vi "NXT_HINDBRAIN Get Sensor Data.vi"(3 "_motorCommands":T1={"_rudderCommand"=7, "_propCommand"=7, "_irServoCommand"=7}, 4 "_sensorData":T2, 5 "NXT":T4) -> (1 "_sensorData":T2)   [LabVIEW 2012, in "Tugboat.lvrbt"]
uses:
  Tugboat.lvrbt
  sensorData_t.ctl
  irData_t.ctl
  <vilib>/NXT/Subs/LVHSConnector.ctl
  motorCommands_t.ctl
  <vilib>/NXT/Block Support/NXT_ButtonSelector.ctl
  <vilib>/NXT/Block Support/NXT_InputPort.ctl
  <vilib>/NXT/Block Support/NXT_TimerIndex.ctl
panel:
  # "L\nE\nF\nT"
  # "C\nE\nN\nT\nE\nR"
  # "R\nI\nG\nH\nT"
  # "L\nE\nF\nT"
  # "C\nE\nN\nT\nE\nR"
  # "R\nI\nG\nH\nT"
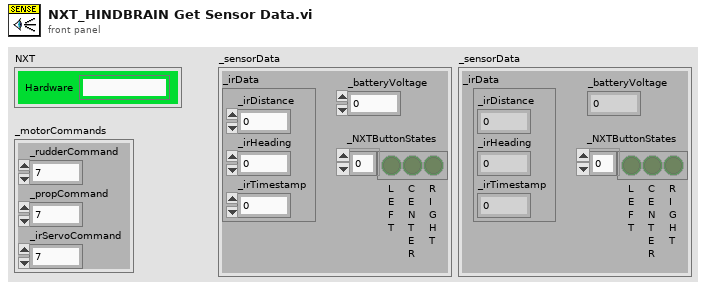
[diagram p1: front panel]
types:
  T1 = typedef "motorCommands_t.ctl" = cluster{"_rudderCommand":i8, "_propCommand":i8, "_irServoCommand":i8}
  T2 = typedef "sensorData_t.ctl" = cluster{"_irData":T3, "_batteryVoltage":i32, "_NXTButtonStates":bool[]}
  T3 = typedef "irData_t.ctl" = cluster{"_irDistance":i32, "_irHeading":i32, "_irTimestamp":u32}
  T4 = typedef "LVHSConnector.ctl" = cluster{"Hardware":string, "Flattened String":string}
  T5 = typedef "NXT_TimerIndex.ctl" = u8
  T6 = typedef "NXT_InputPort.ctl" = u8
  T7 = typedef "NXT_ButtonSelector.ctl" = u16
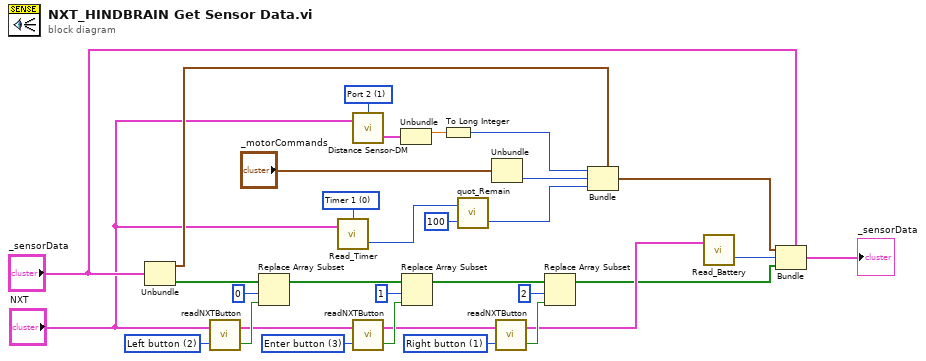
[diagram p0: block diagram]
diagram:
  w7 = T5 0 items=["Timer 1", "Timer 2", "Timer 3"] ("Timer (Timer 1)")
  w13 = T6 1 items=["Port 1", "Port 2", "Port 3", "Port 4"] ("Input Port")
  w19 = T7 1 items=["Enter button"=3, "Left button"=2, "Right button"=1] ("Button (Enter button)")
  w22 = T7 3 items=["Enter button"=3, "Left button"=2, "Right button"=1] ("Button (Enter button)")
  w26 = T7 2 items=["Enter button"=3, "Left button"=2, "Right button"=1] ("Button (Enter button)")
  n1 = Unbundle("_sensorData") -> ("_irData"=w11:T3, "_NXTButtonStates"=w29:bool[])  [unwired: 1 out]
  n2 = call <vilib>:"readNXTButton.vi"("Button (Enter button)"=w26, "NXT"="NXT") -> ("Yes/No"=w27:bool, "NXT"=w18:T4)  [unwired: 1 in]
  n3 = Replace Array Subset(array=w29, new element=w27, index=0) -> (w23:bool[])
  n4 = call <vilib>:"Read_Timer.vi"("NXT"="NXT", "Timer (Timer 1)"=w7) -> ("Value (msec)"=w3:u32)  [unwired: 1 in, 1 out]
  n5 = call "Distance Sensor-DM.vi"("NXT"="NXT", "Input Port"=w13) -> ("Output of Distance Sensor"=w12:cluster{"Distance Value":ext, "Status":bool})  [unwired: 1 in, 1 out]
  n6 = call <vilib>:"readNXTButton.vi"("Button (Enter button)"=w22, "NXT"=w18) -> ("Yes/No"=w24:bool, "NXT"=w17:T4)  [unwired: 1 in]
  n7 = Unbundle(w12) -> ("Distance Value"=w10:ext)  [unwired: 1 out]
  n8 = Replace Array Subset(array=w23, new element=w24, index=1) -> (w16:bool[])
  n9 = To Long Integer(number=w10) -> (32bit integer=w9:i32)
  n10 = call <vilib>:"quot_Remain.vi"("y"=100, "x"=w3) -> ("floor(x/y)"=w1:i32)  [unwired: 1 out]
  n11 = Unbundle("_motorCommands") -> ("_irServoCommand"=w5:i8)  [unwired: 2 out]
  n12 = call <vilib>:"readNXTButton.vi"("Button (Enter button)"=w19, "NXT"=w17) -> ("Yes/No"=w20:bool, "NXT"=w15:T4)  [unwired: 1 in]
  n13 = Replace Array Subset(array=w16, new element=w20, index=2) -> (w14:bool[])
  n14 = Bundle(cluster=w11, "_irDistance"=w9, "_irHeading"=w5, "_irTimestamp"=w1) -> (w6:T3)
  n15 = call <vilib>:"Read_Battery.vi"("NXT"=w15) -> ("millivolts"=w30:i32)  [unwired: 2 in, 1 out]
  n16 = Bundle(cluster="_sensorData", "_irData"=w6, "_batteryVoltage"=w30, "_NXTButtonStates"=w14) -> (→"_sensorData":T2)
